vi "Terminate Test.vi"(8 "error in (no error)":errorcluster, 11 "TestBench in":refnum<class "TestBench.lvclass">) -> (0 "error out":errorcluster, 3 "TestBench out":refnum<class "TestBench.lvclass">)   [LabVIEW 2019, in "TestBench.lvlib" / "TestBench.lvclass"]
uses:
  TestBench.lvclass
  TestBench.lvclass/TestBench.ctl
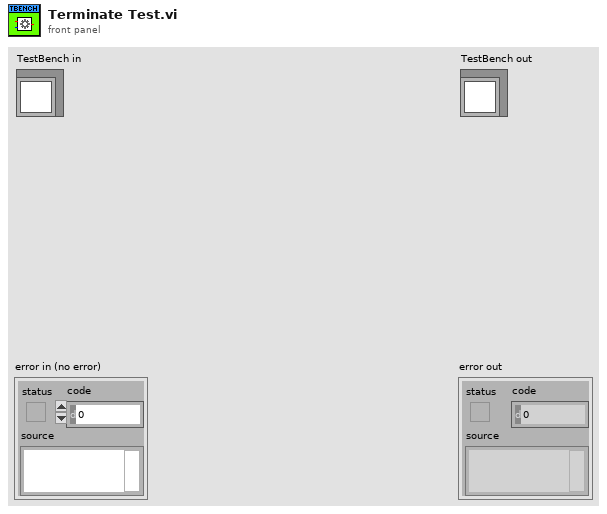
[diagram p1: front panel]
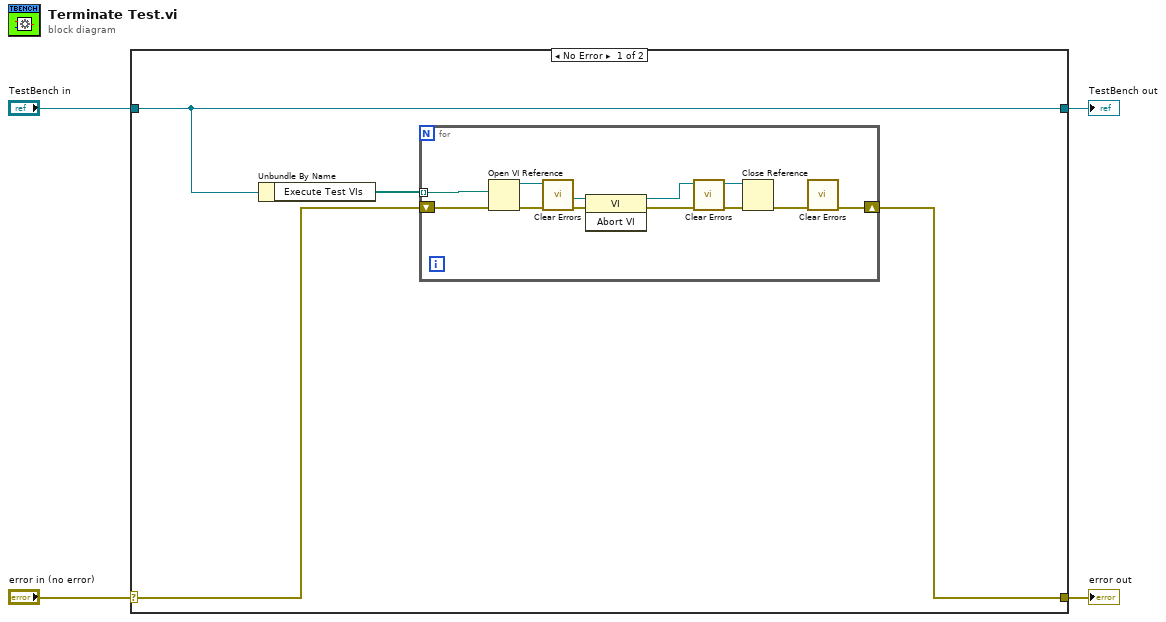
[diagram p0: block diagram]
diagram:
  n1 = case shown="No Error" "error in (no error)" {
    selector: "error in (no error)" -> [w6 w20]
    tunnel: [w5 w20] -> w3
    tunnel: [w8 w19] -> w1
    tunnel: "TestBench in" -> [w8 w19]
    frame No Error {
      n2 = Unbundle By Name(w8) -> ("Execute Test VIs"=w7:path[])
      n3 = for {
        tunnel: w7 -> [w14] mode=indexing
        shift-right: [w9] -> w5
        shift-left: w6 -> [w11]
        n4 = Open VI Reference(vi path=w14, error in (no error)=w11) -> (vi reference=w15:refnum<vi>, error out=w18:errorcluster)  [unwired: 4 in]
        n5 = call <vilib>:"Clear Errors.vi"("error in (no error)"=w18) -> ("error out"=w10:errorcluster)  [unwired: 5 in, 1 out]
        n6 = invoke on="Invoke Node" class="VI" method="Abort VI"(reference=w15, error in=w10) -> (reference out=w17:refnum<vi>, error out=w16:errorcluster)  [unwired: 1 in, 1 out]
        n7 = call <vilib>:"Clear Errors.vi"("error in (no error)"=w16) -> ("error out"=w13:errorcluster)  [unwired: 5 in, 1 out]
        n8 = Close Reference(reference=w17, error in (no error)=w13) -> (error out=w12:errorcluster)
        n9 = call <vilib>:"Clear Errors.vi"("error in (no error)"=w12) -> ("error out"=w9:errorcluster)  [unwired: 5 in, 1 out]
      }
    }
    frame Error {
    }
  }
  "error out" <- w3
  "TestBench out" <- w1
